vi "read_data_feed_mt_connect (SubVI).vi"(8 "error in (no error)":errorcluster, 11 "URL":string="http://amrcadp:5000/current?&path=//") -> (0 "error out":errorcluster, 3 "appended array":dbl[](array[numeric]))   [LabVIEW 2017]
uses:
  <vilib>/xml/Load XML String.vi
  <vilib>/xml/Close Reference(Node).vi
  <vilib>/addons/internet/NI_InternetTK_Core_VIs.lvlib
  <vilib>/xml/NI_XML.lvlib
  <resource>/objmgr/DOMUserDefRef.rc
panel:
  out "concatenated string":string
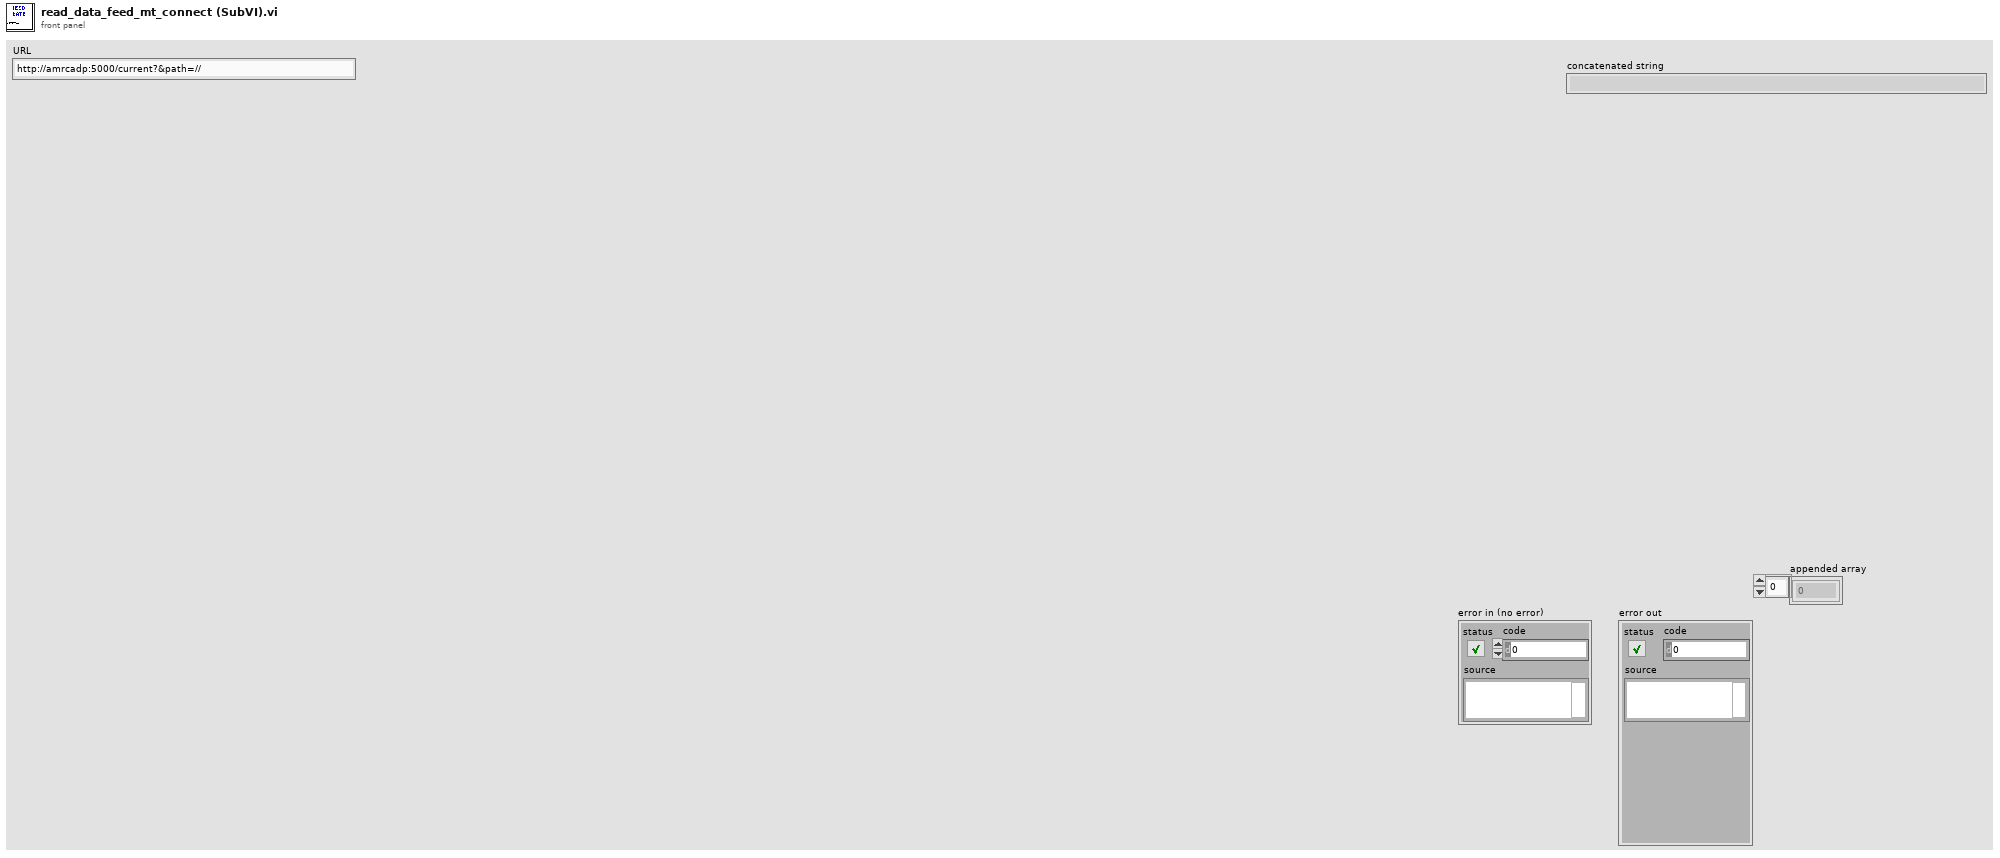
[diagram p1: front panel]
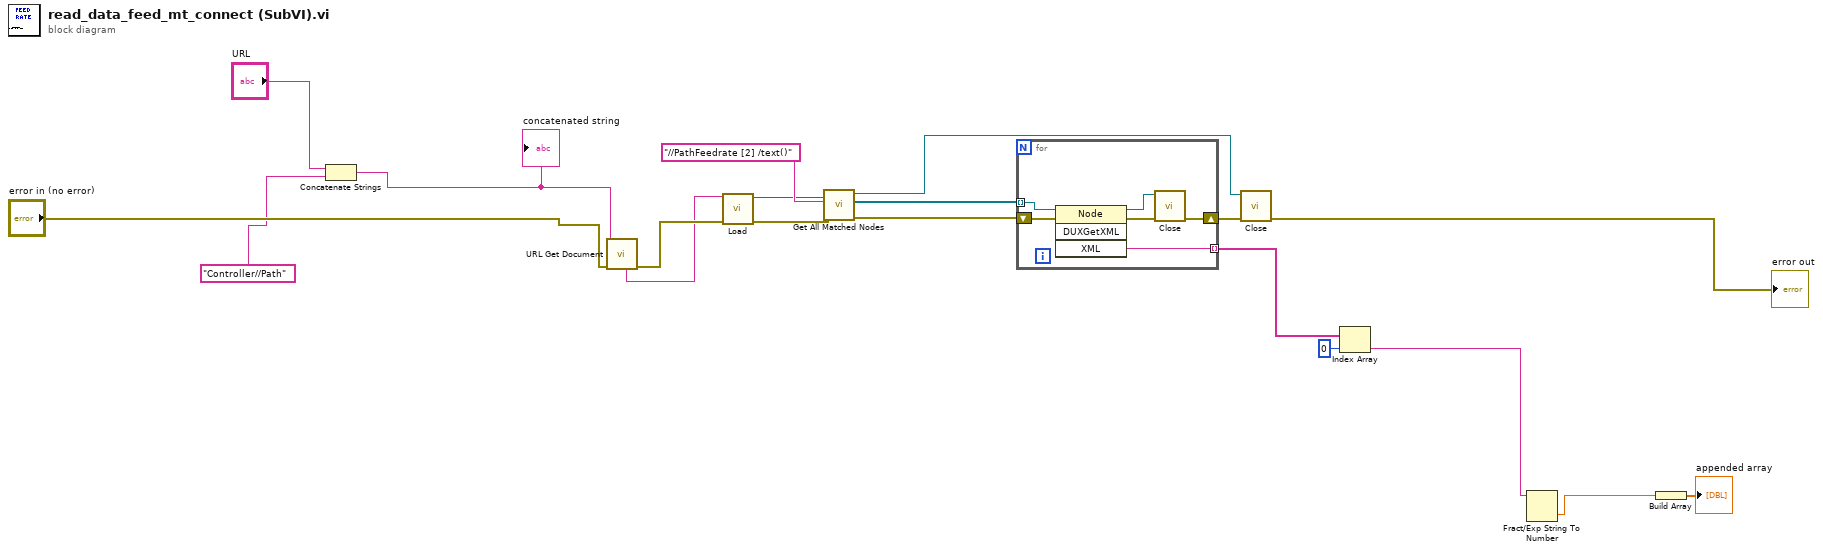
[diagram p0: block diagram]
diagram:
  n1 = Concatenate Strings("URL", "Controller//Path" ("URL")) -> (w1:string)
  "concatenated string" <- w1
  n2 = call <vilib>:"URL Get Document.vi"("error in (no error)"="error in (no error)", "URL"=w1) -> ("error out"=w17:errorcluster, "content"=w15:string)  [unwired: 5 in, 3 out]
  n3 = call-poly <vilib>:"Load.vi"("XML string"=w15, "error in (no error)"=w17) -> ("DOM document out"=w12:refnum<k20>, "error out"=w13:errorcluster)  [unwired: 11 in, 1 out]
  n4 = call <vilib>:"Get All Matched Nodes.vi"("error in (no error)"=w13, "XPath expression"="//PathFeedrate [2] /text()", "node in"=w12) -> ("error out"=w10:errorcluster, "node result array"=w9:refnum<k20>[], "node out"=w14:refnum<k20>)  [unwired: 6 out]
  n5 = for {
    tunnel: w9 -> [w21] mode=indexing
    shift-right: [w23] -> w11
    shift-left: w10 -> [w22]
    tunnel: [w20] -> w8 mode=indexing
    n6 = invoke on="Invoke Node" class="Node" method="DUXGetXML"(reference=w21, error in=w22) -> (reference out=w24:refnum<k20>, error out=w25:errorcluster, "XML"=w20:string)  [unwired: 2 in, 1 out]
    n7 = call-poly <vilib>:"Close.vi"("error in (no error)"=w25, "node"=w24) -> ("error out"=w23:errorcluster)  [unwired: 7 out]
  }
  n8 = call-poly <vilib>:"Close.vi"("error in (no error)"=w11, "node"=w14) -> ("error out"=→"error out":errorcluster)  [unwired: 7 out]
  n9 = Index Array(array=w8, index=0) -> (element=w6:string)
  n10 = Fract/Exp String To Number(string=w6) -> (number=w5:dbl)  [unwired: 3 in, 1 out]
  n11 = Build Array(w5) -> (→"appended array":dbl[])
